vi "Temperature_Regulation.vi"() -> ()   [LabVIEW 2015]
uses:
  Downloads/K8055D.dll
panel:
  out "analog1":dbl
  out "Fan activated":bool
  out "temperature":dbl
  out "Analog2":dbl
  in  "card":dbl
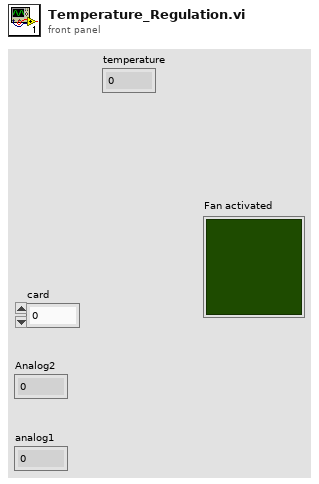
[diagram p1: front panel]
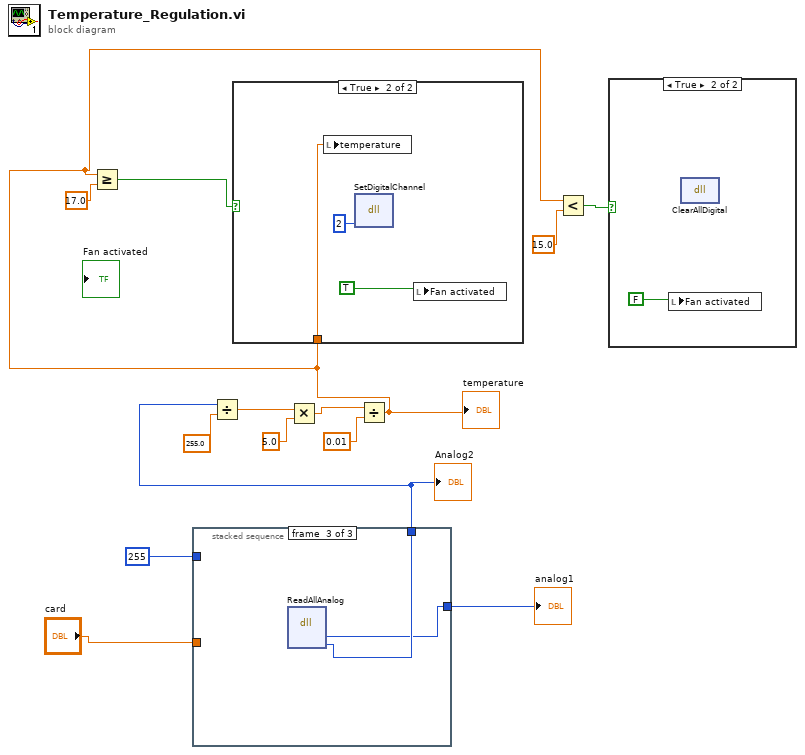
[diagram p0: block diagram]
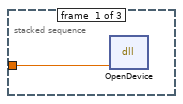
[diagram p4: hidden frame]
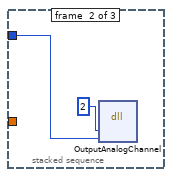
[diagram p5: hidden frame]
diagram:
  n1 = stacked-sequence {
    tunnel: "card" -> [w15 _ _]
    tunnel: [_ _ w19] -> w12
    tunnel: [_ _ w18] -> w5
    tunnel: 255 ("valeur dac2") -> [_ w16 _]
    frame #0 {
      n2 = dll-call lib="C:/Users/g60731/Downloads/K8055D.dll" fn="OpenDevice"("entry card"=w15) -> ()  [unwired: 5 in, 2 out]
    }
    frame #1 {
      n3 = dll-call lib="C:/Users/g60731/Downloads/K8055D.dll" fn="OutputAnalogChannel"("canal dac"=2, "valeur dac2"=w16) -> ()  [unwired: 6 in, 2 out]
    }
    frame #2 {
      n4 = dll-call lib="C:/Users/g60731/Downloads/K8055D.dll" fn="ReadAllAnalog"() -> ("arg1"=w18:i32, "arg2"=w19:i32)  [unwired: 6 in, 2 out]
    }
  }
  "Analog2" <- w12
  "analog1" <- w5
  n5 = Divide(x=w12, y=255.0) -> (x/y=w10:dbl)
  n6 = Multiply(x=w10, y=5.0) -> (x*y=w8:dbl)
  n7 = Divide(x=w8, y=0.01) -> (x/y=w1:dbl)
  "temperature" <- w1
  n8 = Greater Or Equal?(x=w1, y=17.0) -> (x >= y?=w6:bool)
  n9 = case shown="True" w6 {
    tunnel: w1 -> [_ w20]
    frame False {
    }
    frame True {
      n10 = local write "temperature"(w20) -> ()
      n11 = dll-call lib="C:/Users/g60731/Downloads/K8055D.dll" fn="SetDigitalChannel"("sortie2"=2) -> ()  [unwired: 5 in, 2 out]
      n12 = local write "Fan activated"(TRUE) -> ()
    }
  }
  n13 = Less?(x=w1, y=15.0) -> (x < y?=w3:bool)
  n14 = case shown="True" w3 {
    frame False {
    }
    frame True {
      n15 = local write "Fan activated"(FALSE) -> ()
      n16 = dll-call lib="C:/Users/g60731/Downloads/K8055D.dll" fn="ClearAllDigital"() -> ()  [unwired: 4 in, 2 out]
    }
  }
